vi "Image mesurment.vi"(11 "Error In":errorcluster) -> ()   [LabVIEW 2019]
uses:
  <vilib>/userdefined/High Color/IMAQdx.ctl
  Global.vi
  <vilib>/vision/driver/NI_Vision_Acquisition_Software.lvlib
  <resource>/objmgr/imaqdx.rc
  <vilib>/vision/NI_Vision_Development_Module.lvlib
panel:
  out "Pin Angle 2":T1(graph)
  in  "Set initial":bool
  out "Error Out":errorcluster
  in  "Stop Button":bool
  in  "VideoMode":u32
  out "Pin Angle":dbl(graph)
  out "Angle":dbl
  out "intial":cluster{"X0":sgl, "Y0":sgl}
  in  "Vertex":cluster{"X0":dbl, "Y0":dbl}={"X0"=160.0, "Y0"=0.0}
  out "Object Center":cluster{"X":sgl, "Y":sgl}
  out "Image":T2(plugin-control)
  out "Objects":T3(array[cluster]) {"Aspect Ratio" format="%.2f"; "Orientation" format="%.2f"; "Area" format="%.2f"; "Object Center"."Y" format="%.2f"; "Object Center"."X" format="%.2f"}
  in  "Settings":T4={"Objects"=1, "Threshold"=50, "Reject Border"=FALSE, "Fill Holes"=FALSE, "Min Object Size"=TRUE, "Min Size"=101, "Max Object Size"=FALSE, "Max Size"=100, "Show Search Area"=FALSE, "Show Center"=TRUE, "Show Bounding Box"=TRUE} {"Objects" items=["Bright Objects", "Dark Objects"]; "Threshold" min=1 max=999999999 step=1; "Max Size" min=1 max=999999999 step=1; "Min Size" min=1 max=999999999 step=1}
  in  "Session In":T5="cam6"
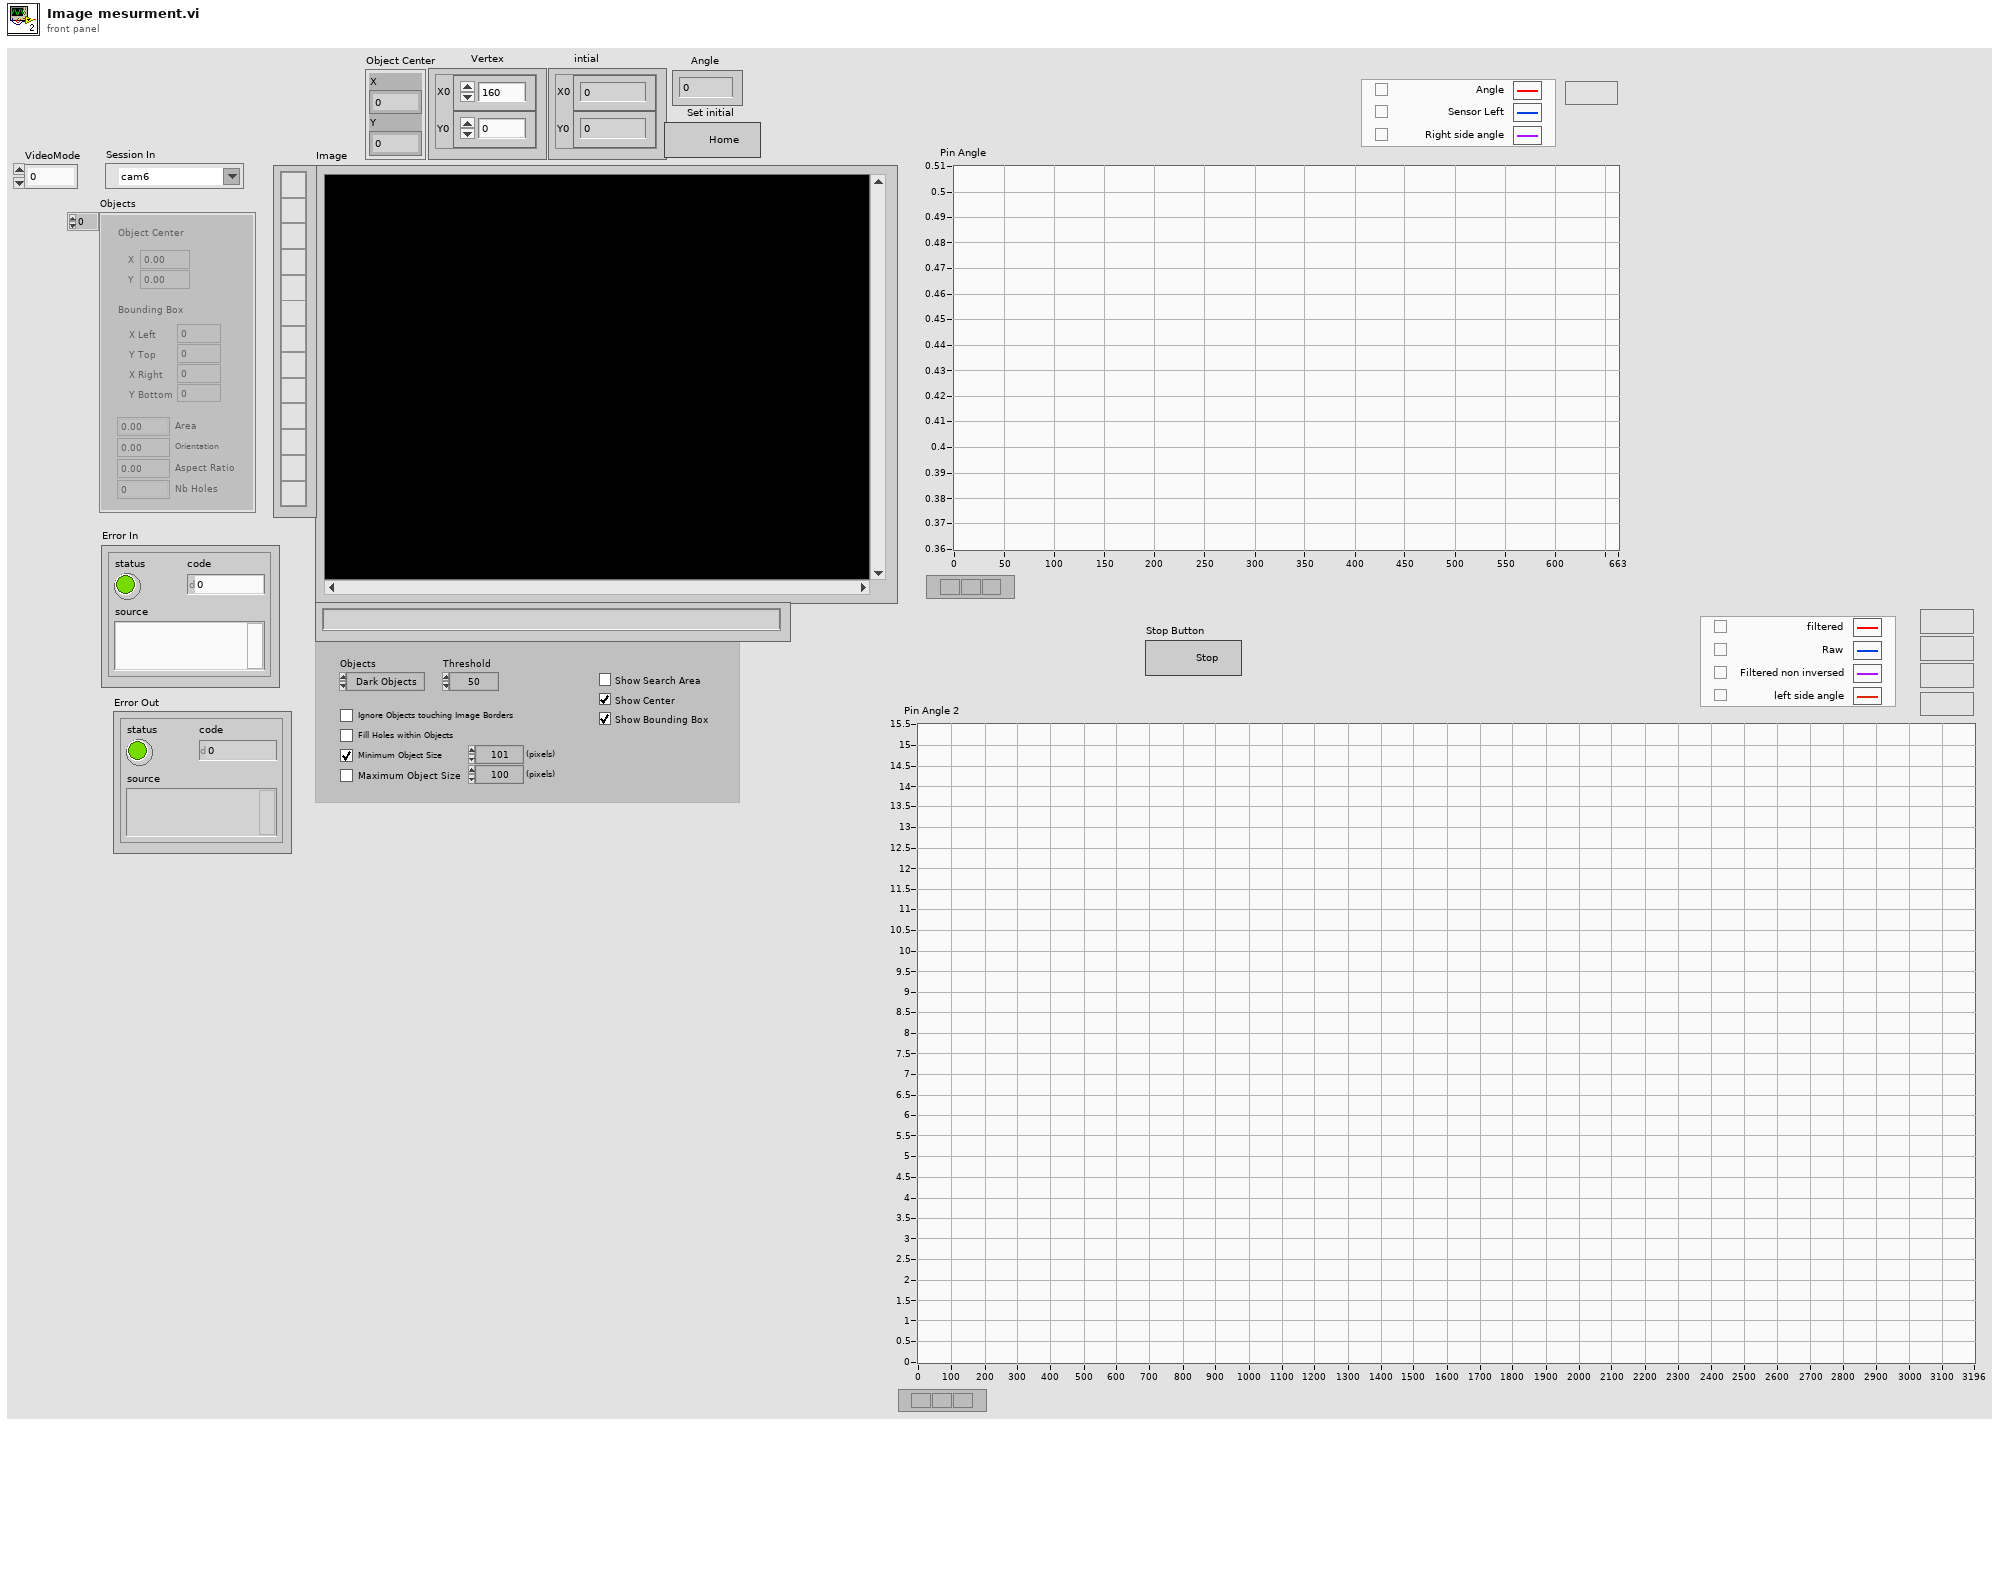
[diagram p1: front panel]
types:
  T1 = cluster{dbl, "Angle modified":dbl, "yf":dbl, "Angle raw":dbl}
  T2 = typedef "IMAQ Image.ctl" = refnum<image>
  T3 = cluster{"Object Center":cluster{"X":sgl, "Y":sgl}, "Bounding Box":cluster{"X Left":i32, "Y Top":i32, "X Right":i32, "Y Bottom":i32}, "Area":sgl, "Orientation":sgl, "Aspect Ratio":sgl, "Nb Holes":i32}[]
  T4 = cluster{"Objects":u16, "Threshold":i32, "Reject Border":bool, "Fill Holes":bool, "Min Object Size":bool, "Min Size":i32, "Max Object Size":bool, "Max Size":i32, "Show Search Area":bool, "Show Center":bool, "Show Bounding Box":bool}
  T5 = typedef "IMAQdx.ctl" = refnum<k21>
  T6 = cluster{"yf":dbl, "Angle modified":dbl, "Angle raw":dbl, "yf":dbl}[]
  T7 = cluster{"Angle":dbl, "Double":dbl, "Double":dbl}[]
  T8 = typedef "IMAQ Rectangle" = cluster{"Left":i32, "Top":i32, "Right":i32, "Bottom":i32, "Rotation":dbl}
  T9 = typedef "Image Type" = u32
  T10 = cluster{"Object Center":cluster{"X":sgl, "Y":sgl}, "Bounding Box":cluster{"X Left":i32, "Y Top":i32, "X Right":i32, "Y Bottom":i32}, "Area":sgl, "Orientation":sgl, "Aspect Ratio":sgl, "Nb Holes":i32}
  T11 = cluster{"yf":dbl, "Angle modified":dbl, "yf":dbl, "Angle raw":dbl}
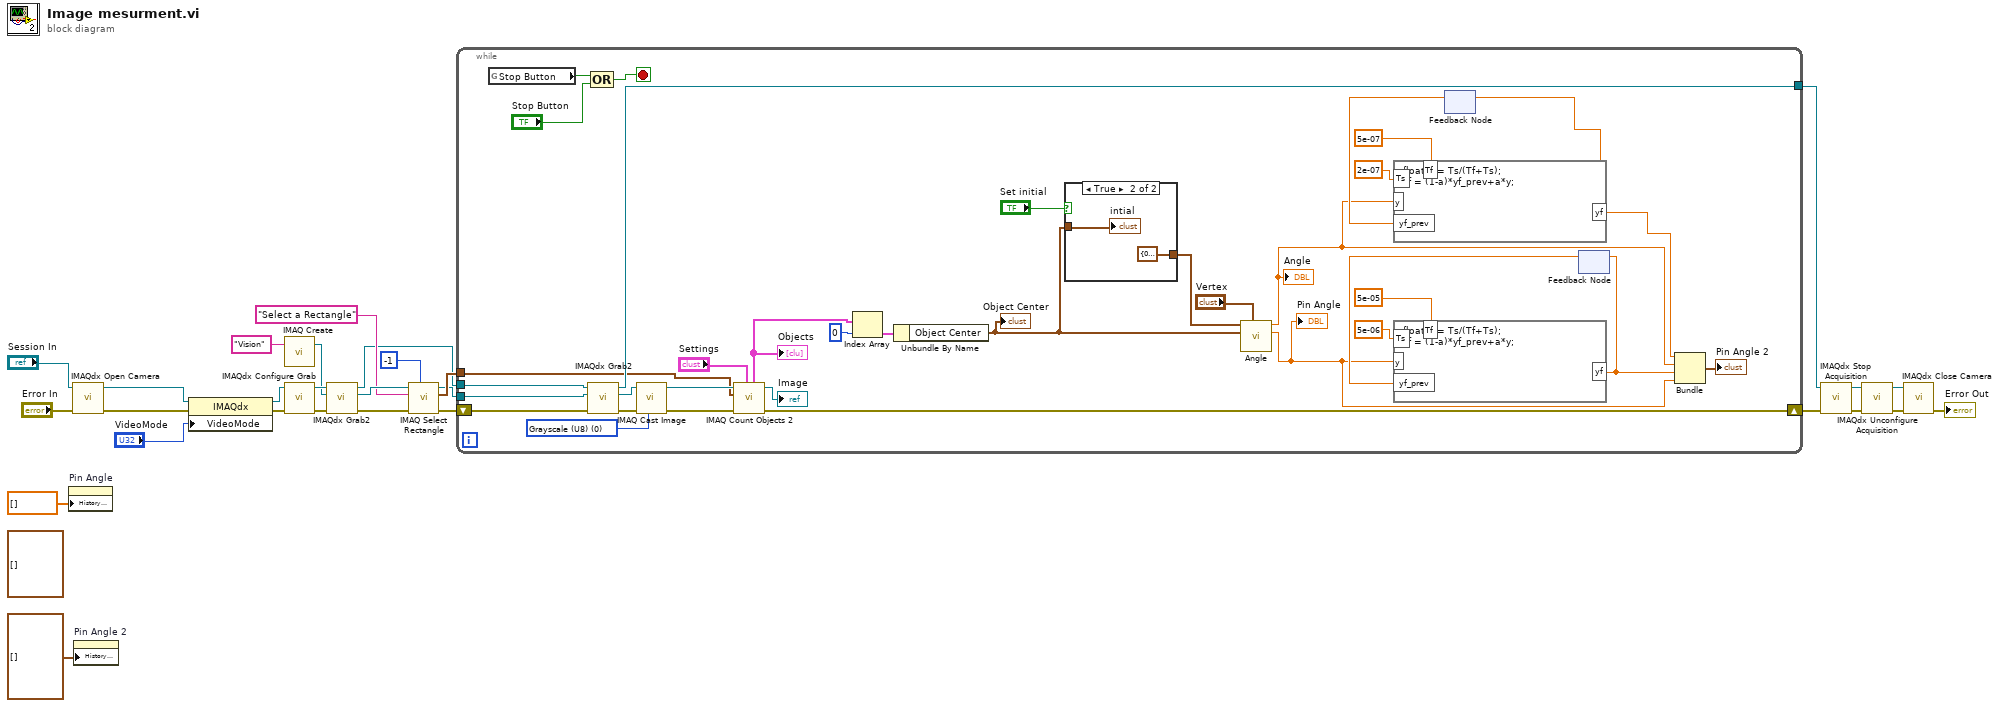
[diagram p0: block diagram]
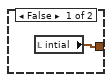
[diagram p2: hidden frame]
diagram:
  (unwired) T7 [] ("History Data")
  n1 = property on="Pin Angle" class="WFChart (strict)"("History Data"=dbl[] []) -> ()  [unwired: 2 in, 2 out]
  n2 = call <vilib>:"IMAQdx Open Camera.vi"("error in"="Error In", "Session In"="Session In") -> ("error out"=w14:errorcluster, "Session Out"=w15:T5)  [unwired: 8 in]
  n3 = property on="Pin Angle 2" class="WFChart (strict)"("History Data"=T6 []) -> ()  [unwired: 2 in, 2 out]
  n4 = property class="IMAQdx"(reference=w15, error in=w14, "VideoMode"="VideoMode") -> (reference out=w13:T5, error out=w12:errorcluster)
  n5 = call "IMAQ Create"("Image Name"="Vision") -> ("New Image"=w24:T2)  [unwired: 4 in, 1 out]
  n6 = call <vilib>:"IMAQdx Configure Grab.vi"("error in"=w12, "Session In"=w13) -> ("error out"=w23:errorcluster, "Session Out"=w28:T5)  [unwired: 8 in]
  n7 = call <vilib>:"IMAQdx Grab2.vi"("error in"=w23, "Image In"=w24, "Session In"=w28) -> ("error out"=w22:errorcluster, "Image Out"=w27:T2, "Session Out"=w4:T5)  [unwired: 5 in, 1 out]
  n8 = call "IMAQ Select Rectangle"("Window Number (0...15)"=-1, "error in (no error)"=w22, "Prompt"="Select a Rectangle", "Image In"=w27) -> ("error out"=w7:errorcluster, "Rectangle"=w5:T8, "Image Out (duplicate)"=w3:T2)  [unwired: 4 in, 1 out]
  n9 = while {
    tunnel: w5 -> [w46]
    tunnel: w3 -> [w44]
    shift-right: [w49] -> w8
    shift-left: w7 -> [w48]
    tunnel: w4 -> [w45]
    tunnel: [w47] -> w6
    stop <- w43 stop-if-true
    w59 = T9 0 items=["Grayscale (U8)", "Grayscale (I16)", "Grayscale (SGL)", "Complex (CSG)", "RGB (U32)", "HSL (U32)", "RGB (U64)", "Grayscale (U16)"] ("Image Type")
    n10 = global read "Global.vi" "Stop Button"() -> (w61:bool)
    n11 = call <vilib>:"IMAQdx Grab2.vi"("error in"=w48, "Image In"=w44, "Session In"=w45) -> ("error out"=w55:errorcluster, "Image Out"=w54:T2, "Session Out"=w47:T5)  [unwired: 5 in, 1 out]
    n12 = Compound Arithmetic op=OR(w61, "Stop Button") -> (w43:bool)
    n13 = call "IMAQ Cast Image"("Image Type"=w59, "error in (no error)"=w55, "Image Src"=w54) -> ("error out"=w56:errorcluster, "Image Dst Out"=w57:T2)  [unwired: 7 in]
    n14 = call "IMAQ Count Objects 2"("Settings"="Settings", "error in (no error)"=w56, "Search Rect (entire image)"=w46, "Image"=w57) -> ("error out"=w49:errorcluster, "Image Out"=→"Image":T2, "Objects"=w51:T3)  [unwired: 3 in, 2 out]
    "Objects" <- w51
    n15 = Index Array(array=w51, index=0) -> (element=w53:T10)
    n16 = Unbundle By Name(w53) -> ("Object Center"=w42:cluster{"X":sgl, "Y":sgl})
    "Object Center" <- w42
    n17 = case shown="True" "Set initial" {
      tunnel: w42 -> [_ w65]
      tunnel: [w63 cluster{"X0":sgl, "Y0":sgl} {"X0"=0.0, "Y0"=0.0} ("intial")] -> w40
      frame False {
        n18 = local read "intial"() -> (w63:cluster{"X0":sgl, "Y0":sgl})
      }
      frame True {
        "intial" <- w65
      }
    }
    n19 = call "Angle.vi"("Vertex"="Vertex", "Object"=w42, "initial"=w40) -> ("Angle raw"=w29:dbl, "Angle modified"=w35:dbl)  [unwired: 7 in]
    "Angle" <- w35
    "Pin Angle" <- w29
    n20 = feedback #1() -> (w39:dbl)  [unwired: 1 in]
    n21 = formula code="float a = Ts/(Tf+Ts);\nyf = (1-a)*yf_prev+a*y;"("Tf"=5e-07 ("input variable"), "Ts"=2e-07 ("input variable"), "y"=w35, "yf_prev"=w39) -> ("yf"=w30:dbl)
    n22 = feedback-in #1(w30) -> ()
    n23 = feedback #2() -> (w32:dbl)  [unwired: 1 in]
    n24 = formula code="float a = Ts/(Tf+Ts);\nyf = (1-a)*yf_prev+a*y;"("Tf"=5e-05 ("input variable"), "Ts"=5e-06 ("input variable"), "y"=w29, "yf_prev"=w32) -> ("yf"=w31:dbl)
    n25 = feedback-in #2(w31) -> ()
    n26 = Bundle("yf"=w30, "Angle modified"=w35, "yf"=w31, "Angle raw"=w29) -> (→"Pin Angle 2":T11)  [unwired: 1 in]
  }
  n27 = call <vilib>:"IMAQdx Stop Acquisition.vi"("error in"=w8, "Session In"=w6) -> ("error out"=w19:errorcluster, "Session Out"=w18:T5)  [unwired: 8 in]
  n28 = call <vilib>:"IMAQdx Unconfigure Acquisition.vi"("error in"=w19, "Session In"=w18) -> ("error out"=w17:errorcluster, "Session Out"=w16:T5)  [unwired: 8 in]
  n29 = call <vilib>:"IMAQdx Close Camera.vi"("error in"=w17, "Session In"=w16) -> ("error out"=→"Error Out":errorcluster)  [unwired: 9 in]
